vi "Progress Counter.vi"(8 "y":dbl, 9 "x":dbl, 11 "Map size (Pixels)":dbl) -> (1 "Progress":dbl(slide) scale=0.0..100.0, 3 "Loop counter":dbl)   [LabVIEW 2022 SP3]
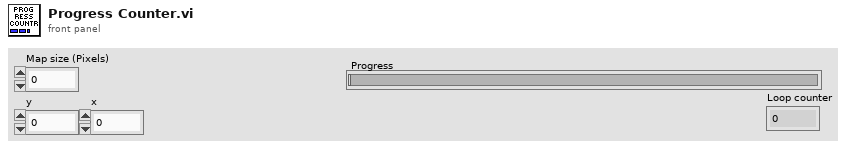
[diagram p1: front panel]
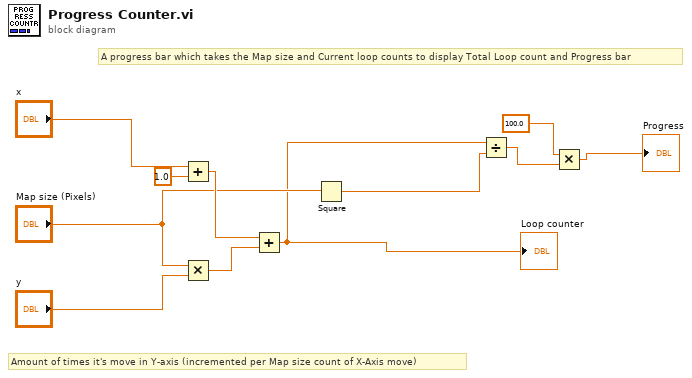
[diagram p0: block diagram]
diagram:
  # "Amount of times it's move in Y-axis (incremented per Map size count of X-Axis move)"
  # "A progress bar which takes the Map size and Current loop counts to display Total Loop count and Progress bar"
  n1 = Add(x="x", y=1.0) -> (x+y=w7:dbl)
  n2 = Multiply(x="Map size (Pixels)", y="y") -> (x*y=w8:dbl)
  n3 = Add(x=w7, y=w8) -> (x+y=w4:dbl)
  "Loop counter" <- w4
  n4 = Square(x="Map size (Pixels)") -> (x^2=w5:dbl)
  n5 = Divide(x=w4, y=w5) -> (x/y=w3:dbl)
  n6 = Multiply(x=100.0, y=w3) -> (x*y=→"Progress":dbl)
